vi "Launch Autocomplete Handler.vi"(7 "LstBox Refnum (Popup)":refnum<vi>, 8 "error in (no error)":errorcluster, 9 "Height (200)":i16=200, 10 "Initial Options (Empty)":string[](array[string]), 11 "Str Refnum":refnum<vi>) -> (0 "error out":errorcluster, 2 "New Options Event":refnum<user-event>, 3 "Stop Event":refnum<user-event>)   [LabVIEW 2020, in "FlexBlocks.lvlib"]
uses:
  FlexBlocks.lvlib
  Autocomplete UI.vi
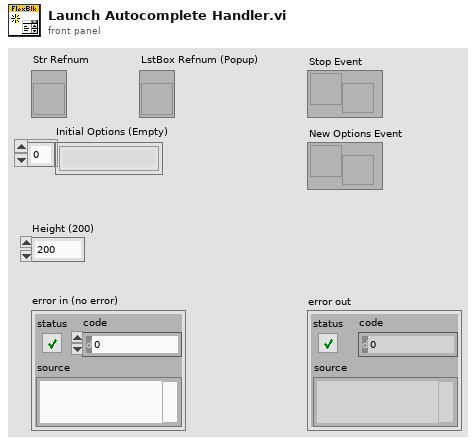
[diagram p1: front panel]
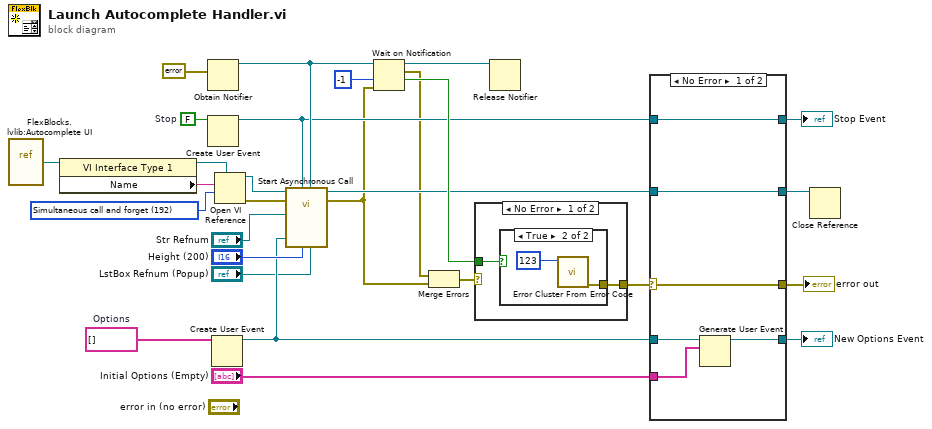
[diagram p0: block diagram]
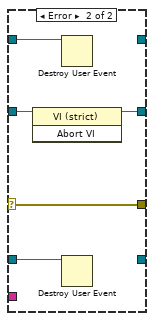
[diagram p4: hidden frame]
diagram:
  w20 = string[] []  # Options
  w24 = 192 items=["Record modifications"=1, "Open templates for editing"=2, "Prompt user to save"=4, "Prepare for reentrant run"=8, "Prompt to find missing subVIs"=16, "Hide loading dialog box"=32, "Enable simultaneous calls"=64, "Prepare to call and forget"=128, "Simultaneous call and forget"=192, "Prepare to call and collect"=256, "Simultaneous call and collect"=320]
  w28 = FALSE  # Stop
  n1 = vi-ref "FlexBlocks.lvlib:Autocomplete UI.vi"() -> (w22:refnum<vi>)
  n2 = property class="VI Interface Type 1"(reference=w22) -> (reference out=w25:refnum<vi>, "Name"=w23:string)  [unwired: 1 in, 1 out]
  n3 = Obtain Notifier(notification data type=errorcluster {"status"=FALSE, "code"=0, "source"=""} ("error constant")) -> (notifier out=w17:refnum<notifier>)  [unwired: 3 in, 2 out]
  n4 = Create User Event(user event datatype=w28) -> (user event=w8:refnum<user-event>)  [unwired: 1 in, 1 out]
  n5 = Create User Event(user event datatype=w20) -> (user event=w13:refnum<user-event>)  [unwired: 1 in, 1 out]
  n6 = Open VI Reference(type specifier VI Refnum (for type only)=w25, vi path=w23, options=w24) -> (vi reference=w27:refnum<vi>, error out=w26:errorcluster)  [unwired: 3 in]
  n7 = call-by-ref "Start Asynchronous Call"(reference=w27, error in=w26, "LstBox Refnum"="LstBox Refnum (Popup)", "Ready Notifier"=w17, "Height (200)"="Height (200)", "Stop Event"=w8, "Options"=w13, "Str Refnum"="Str Refnum") -> (reference out=w11:refnum<vi>, error out=w2:errorcluster)  [unwired: 6 in]
  n8 = Wait on Notification(notifier=w17, timeout in ms (-1)=-1, error in (no error)=w2) -> (notifier out=w15:refnum<notifier>, notification=w4:errorcluster, timed out?=w14:bool)  [unwired: 1 in, 1 out]
  n9 = Merge Errors(w4, w2) -> (w3:errorcluster)
  n10 = case shown="No Error" w3 {
    selector: w3 -> [_ w33]
    tunnel: w14 -> [w30 _]
    tunnel: [w29 w33] -> w12
    frame No Error {
      n11 = case shown="True" w30 {
        tunnel: [_ w31] -> w29
        frame False {
        }
        frame True {
          n12 = call <vilib>:"Error Cluster From Error Code.vi"("error code (0)"=123) -> ("error out"=w31:errorcluster)  [unwired: 8 in]
        }
      }
    }
    frame Error {
    }
  }
  n13 = Release Notifier(notifier=w15) -> ()  [unwired: 2 in, 3 out]
  n14 = case shown="No Error" w12 {
    selector: w12 -> [w37 w40]
    tunnel: w13 -> [w36 w41]
    tunnel: w11 -> [w39 w44]
    tunnel: [w39 w43] -> w10
    tunnel: [w38 _] -> w9
    tunnel: w8 -> [w38 w42]
    tunnel: [w34 _] -> w7
    tunnel: [w37 w40] -> w6
    tunnel: "Initial Options (Empty)" -> [w35 _]
    frame No Error {
      n15 = Generate User Event(user event=w36, event data cluster=w35) -> (user event out=w34:refnum<user-event>)  [unwired: 2 in, 1 out]
    }
    frame Error {
      n16 = invoke class="VI (strict)" method="Abort VI"(reference=w44) -> (reference out=w43:refnum<vi>)  [unwired: 2 in, 2 out]
      n17 = Destroy User Event(user event=w42) -> ()  [unwired: 1 in, 1 out]
      n18 = Destroy User Event(user event=w41) -> ()  [unwired: 1 in, 1 out]
    }
  }
  "Stop Event" <- w9
  "New Options Event" <- w7
  "error out" <- w6
  n19 = Close Reference(reference=w10) -> ()  [unwired: 1 in, 1 out]
